vi "Convert Waveform to Arrays.vi"(11 "Waveform In":waveform(dbl)) -> (2 "X Values (Seconds)":dbl[](array[numeric]), 3 "Y Values (Voltage)":dbl[](array[numeric]))   [LabVIEW 2021]
doc: "Converts the dataset from a waveform, into two sets of arrays (Voltage & Time[Seconds])."
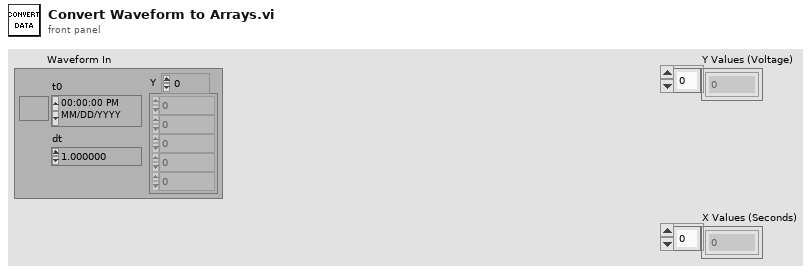
[diagram p1: front panel]
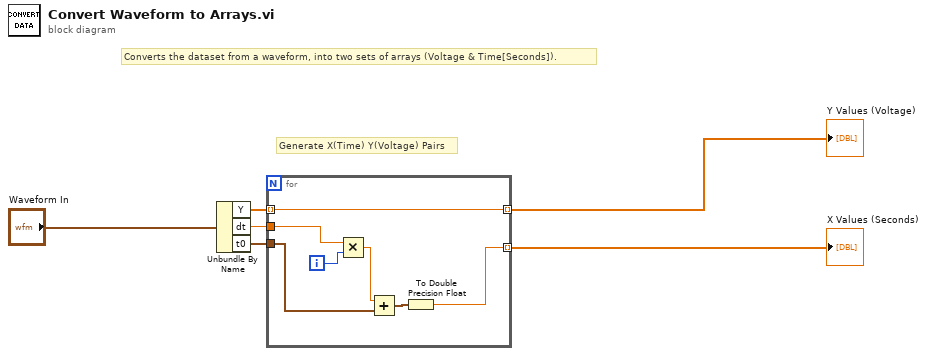
[diagram p0: block diagram]
diagram:
  # "Converts the dataset from a waveform, into two sets of arrays (Voltage & Time[Seconds])."
  # "Generate X(Time) Y(Voltage) Pairs"
  n1 = Unbundle By Name("Waveform In") -> ("Y"=w5:dbl[], "dt"=w4:dbl, "t0"=w1:timestamp)
  n2 = for {
    tunnel: w5 -> [w12] mode=indexing
    tunnel: w4 -> [w10]
    tunnel: [w7] -> w2 mode=indexing
    tunnel: [w12] -> w3 mode=indexing
    tunnel: w1 -> [w11]
    i -> [w13]
    n3 = Multiply(x=w10, y=w13) -> (x*y=w8:dbl)
    n4 = Add(x=w8, y=w11) -> (x+y=w9:timestamp)
    n5 = To Double Precision Float(number=w9) -> (double precision float=w7:dbl)
  }
  "Y Values (Voltage)" <- w3
  "X Values (Seconds)" <- w2
